vi "Request Plugin Loader Stop.vi"(8 "error in (no error)":errorcluster, 10 "Plugin Loader Name":string, 11 "CIFPluginManager in":refnum<class "CIFPluginManager.lvclass">) -> (0 "error out":errorcluster, 3 "gRPC ID":T1)   [LabVIEW 2021, in "CIFPluginManager.lvclass"]
uses:
  CIFPluginManager.lvclass
  CIFPluginManager.lvclass/CIFPluginManager.ctl
  <vilib>/Utility/miscctls.llb/LVMapReplaceAction.ctl
  CIFCore/Common/CIFCoreCommon.lvlib
  CIFCore/Common/Typedef/Errors.ctl
  <vilib>/CIF Foundation/CIF Utilities/Time/Time_CIF_U.lvlib
  <vilib>/gRPC/LabVIEW gRPC Library/Shared/grpcId.ctl
  <vilib>/gRPC/LabVIEW gRPC Library/grpc-lvsupport-release.lvlib
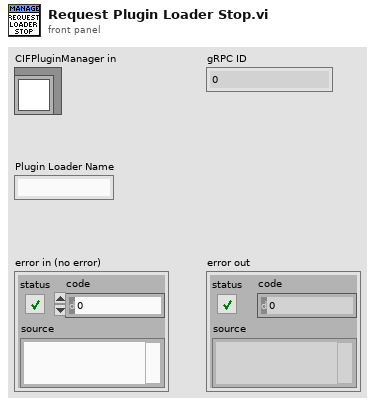
[diagram p1: front panel]
types:
  T1 = typedef "grpc-lvsupport-release.lvlib/grpcId.ctl" = u64
  T2 = typedef "LVMapReplaceAction.ctl" = enum32{"Modify Entry only if found", "Add or Modify Entry", "Delete Entry"}
  T3 = typedef "CIFCoreCommon.lvlib/Errors.ctl" = enum16{"Invalid Clock ID", "Long Sleep", "gRPC Server Not Found", "Config Parse", "Timestamp Wrap", "Delayed Execution", "Duplicate Channel", "Missing Channel", "Incorrect Type", "Flatten Error", "Unflatten Data", "Unique Name", "Plugin Not Found", "Plugin Type Not Found", "Plugin Version Not Found", "Manager Not Found", "Numerical Issue", "Time Jump", "Clock ID Match", "Channel Length", "Plugin Connection", "gRPC Server Connection", "PPL Name Match", "Build", "Config Log Parse", "Plugin Load", "UI Subpanel Load", "Python Name", "Invalid Name", "Unable to Change Ch Buffer"}
  T4 = typedef "CIFPluginManager.lvclass/Loader Map.ctl" = map{string, T5}
  T5 = typedef "CIFPluginManager.lvclass/Loaders.ctl" = cluster{"Loader Type":T6, "grpc_port":i32, "pid":u32, "gRPC ID":T1, "Load Timestamp":i64, "Unloading":bool, "Ready for removal":bool, "Unload Timestamp":i64}
  T6 = typedef "CIFPluginManager.lvclass/Loader Type.ctl" = enum16{"LabVIEW"}
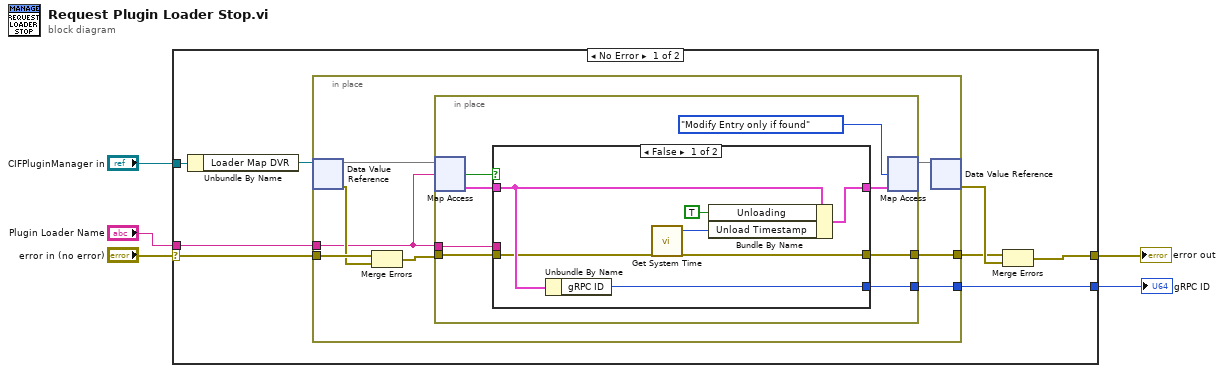
[diagram p0: block diagram]
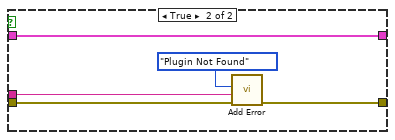
[diagram p2: hidden frame]
diagram:
  n1 = case shown="No Error" "error in (no error)" {
    selector: "error in (no error)" -> [w8 w41]
    tunnel: "CIFPluginManager in" -> [w13 _]
    tunnel: [w10 w41] -> w2
    tunnel: "Plugin Loader Name" -> [w9 _]
    tunnel: [w6 _] -> w1
    frame No Error {
      n2 = Unbundle By Name(w13) -> ("Loader Map DVR"=w12:refnum<data-value>)
      n3 = in-place {
        in-place-border: [w16] -> w7
        in-place-border: w9 -> [w15]
        in-place-border: w8 -> [w19]
        in-place-border: [w14] -> w6
        n4 = in-place-dvr #1(w12) -> (w21:T4, w18:errorcluster)
        n5 = Merge Errors(w19, w18) -> (w17:errorcluster)
        n6 = in-place {
          in-place-border: w17 -> [w28]
          in-place-border: [w26] -> w16
          in-place-border: w15 -> [w23]
          in-place-border: [w22] -> w14
          n7 = in-place-map #2(w21, w15) -> (w29:T5, w25:bool)  [unwired: 1 in]
          n8 = case shown="False" w25 {
            tunnel: w29 -> [w35 w40]
            tunnel: w28 -> [w31 w38]
            tunnel: [w33 w40] -> w27
            tunnel: [w31 w37] -> w26
            tunnel: w23 -> [_ w36]
            tunnel: [w30 _] -> w22
            frame False {
              n9 = Unbundle By Name(w35) -> ("gRPC ID"=w30:T1)
              n10 = call <vilib>:"Get System Time.vi"() -> ("Time (ns)"=w32:i64)  [unwired: 5 in]
              n11 = Bundle By Name(cluster=w35, "Unloading"=TRUE, "Unload Timestamp"=w32) -> (w33:T5)
            }
            frame True {
              n12 = call "Add Error.vi"("error in (no error)"=w38, "String to Append"=w36, "Error"=Errors."Plugin Not Found") -> ("error out"=w37:errorcluster)  [unwired: 8 in]
            }
          }
          n13 = in-place-map #2(w27, LVMapReplaceAction."Modify Entry only if found" ("action")) -> (w20:T4)  [unwired: 2 out]
        }
        n14 = in-place-dvr #1(w20) -> (w11:errorcluster)  [unwired: 1 out]
      }
      n15 = Merge Errors(w7, w11) -> (w10:errorcluster)
    }
    frame Error {
    }
  }
  "error out" <- w2
  "gRPC ID" <- w1
